vi "fft_single.vi"(1 "双边fft":dbl[](graph)) -> (0 "单边fft":dbl[](graph))   [LabVIEW 2022 SP3]
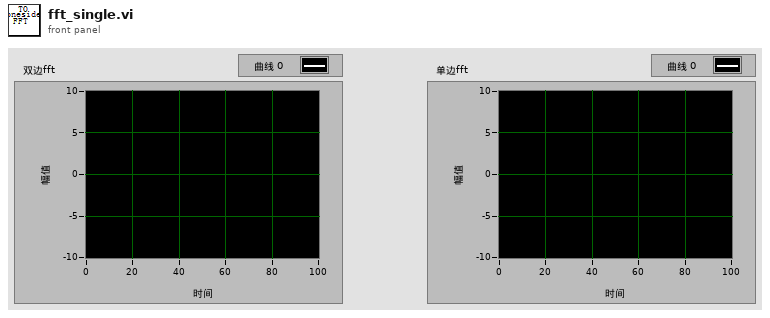
[diagram p1: front panel]
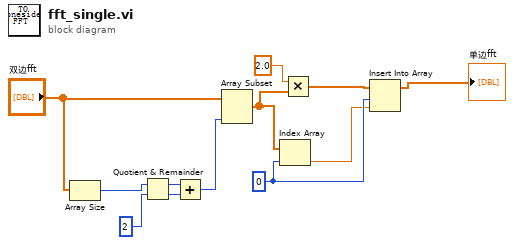
[diagram p0: block diagram]
diagram:
  w3 = 0
  n1 = Array Size(array="双边fft") -> (size(s)=w12:i32)
  n2 = Quotient & Remainder(x=w12, y=2) -> (x-y*floor(x/y)=w9:i32, floor(x/y)=w10:i32)
  n3 = Add(x=w9, y=w10) -> (x+y=w8:i32)
  n4 = Array Subset(array="双边fft", length=w8) -> (w5:dbl[])  [unwired: 1 in]
  n5 = Index Array(array=w5, index=w3) -> (element=w2:dbl)
  n6 = Multiply(x=2.0, y=w5) -> (x*y=w4:dbl[])
  n7 = Insert Into Array(array=w4, index=w3, new element=w2) -> (→"单边fft":dbl[])
